vi "trivial_rep.vi"() -> ()   [LabVIEW 2014]
uses:
  lvnanomsg/nanomsg_context.lvclass
  lvnanomsg/nanomsg_socket.lvclass
panel:
  out "msg":string
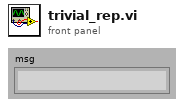
[diagram p1: front panel]
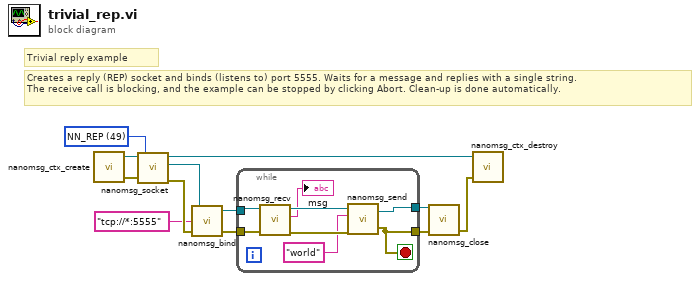
[diagram p0: block diagram]
diagram:
  w8 = 49 items=["NN_WS"=-4, "NN_TCP"=-3, "NN_IPC"=-2, "NN_INPROC"=-1, "NN_SOL_SOCKET"=0, "NN_PAIR"=16, "NN_PUB"=32, "NN_SUB"=33, "NN_REQ"=48, "NN_REP"=49, "NN_PUSH"=80, "NN_PULL"=81, "NN_SURVEYOR"=98, "NN_RESPONDENT"=99, "NN_BUS"=112] ("socket type")
  # "Creates a reply (REP) socket and binds (listens to) port 5555. Waits for a message and replies with a single string.\nThe receive call is blocking, and the example can be stopped by clicking Abort. Clean-up is done automatically."
  # "Trivial reply example"
  n1 = call "nanomsg_ctx_create.vi"() -> ("error out"=w10:errorcluster, "context out"=w9:refnum<class "nanomsg_context.lvclass">)  [unwired: 4 in]
  n2 = call "nanomsg_socket.vi"("error in"=w10, "socket type"=w8, "context in"=w9) -> ("error out"=w12:errorcluster, "socket out"=w11:refnum<class "nanomsg_socket.lvclass">, "context out"=w1:refnum<class "nanomsg_context.lvclass">)  [unwired: 2 in]
  n3 = call "nanomsg_bind.vi"("error in"=w12, "endpoint"="tcp://*:5555", "socket in"=w11) -> ("error out"=w5:errorcluster, "socket out"=w6:refnum<class "nanomsg_socket.lvclass">)  [unwired: 1 in]
  n4 = while {
    tunnel: w6 -> [w19]
    tunnel: w5 -> [w20]
    tunnel: [w14] -> w4
    tunnel: [w13] -> w3
    stop <- w14 stop-if-true
    n5 = call "nanomsg_recv.vi"("error in"=w20, "socket in"=w19) -> ("error out"=w18:errorcluster, "data"=→"msg":string, "socket out"=w17:refnum<class "nanomsg_socket.lvclass">)  [unwired: 3 in, 2 out]
    n6 = call "nanomsg_send.vi"("error in"=w18, "data"="world", "socket in"=w17) -> ("error out"=w14:errorcluster, "socket out"=w13:refnum<class "nanomsg_socket.lvclass">)  [unwired: 1 in]
  }
  n7 = call "nanomsg_close.vi"("error in"=w4, "socket"=w3) -> ("error out"=w2:errorcluster)  [unwired: 3 in]
  n8 = call "nanomsg_ctx_destroy.vi"("error in"=w2, "context in"=w1) -> ()  [unwired: 3 in, 1 out]
